vi "AutonVisionTrack.vi"(3 "Refnum in":refnum<k33>) -> (10 "rt fifo out":refnum<k33>)   [LabVIEW 2014]
uses:
  TeleopCmd.ctl
  CmdFlag.ctl
  VisionInfoCluster.ctl
  AutonCals.vi
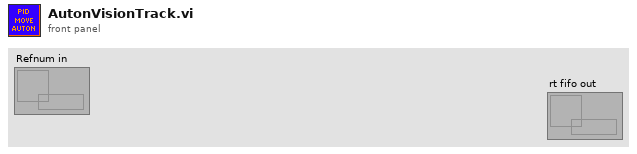
[diagram p1: front panel]
types:
  T1 = typedef "VisionInfoCluster.ctl" = cluster{"X":dbl, "Y":dbl}
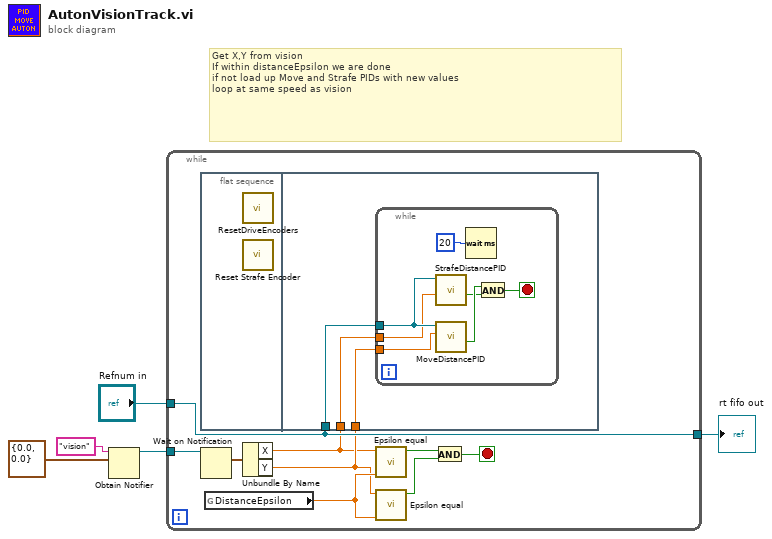
[diagram p0: block diagram]
diagram:
  # "Get X,Y from vision\nIf within distanceEpsilon we are done\nif not load up Move and Strafe PIDs with new values\nloop at same speed as vision"
  n1 = Obtain Notifier(name (unnamed)="vision", notification data type=T1 {"X"=0.0, "Y"=0.0}) -> (notifier out=w3:refnum<notifier>)  [unwired: 2 in, 2 out]
  n2 = while {
    tunnel: w3 -> [w11]
    tunnel: "Refnum in" -> [w8]
    tunnel: [w8] -> w1
    stop <- w12 stop-if-true
    n3 = flat-sequence {
      tunnel: w8 -> [w17]
      tunnel: w7 -> [w16]
      tunnel: w6 -> [w15]
      frame #0 {
        n4 = call "ResetDriveEncoders.vi"() -> ()  [unwired: 12 in]
        n5 = call "Reset Strafe Encoder.vi"() -> ()  [unwired: 12 in]
      }
      frame #1 {
        n6 = while {
          tunnel: w17 -> [w20]
          tunnel: w16 -> [w19]
          tunnel: w15 -> [w18]
          stop <- w24 stop-if-true
          n7 = call "StrafeDistancePID.vi"("Distance"=w18, "Refnum in"=w20) -> ("Boolean"=w22:bool)  [unwired: 7 in, 2 out]
          n8 = call "MoveDistancePID.vi"("Distance"=w19, "Refnum in"=w20) -> ("Boolean"=w23:bool)  [unwired: 7 in, 2 out]
          n9 = Wait (ms)(milliseconds to wait=u32 20) -> ()  [unwired: 1 out]
          n10 = And(x=w23, y=w22) -> (x .and. y?=w24:bool)
        }
      }
    }
    n11 = Wait on Notification(notifier=w11) -> (notification=w10:T1)  [unwired: 3 in, 3 out]
    n12 = global read "AutonCals.vi" "DistanceEpsilon"() -> (w9:dbl)
    n13 = Unbundle By Name(w10) -> ("X"=w6:dbl, "Y"=w7:dbl)
    n14 = call "Epsilon equal.vi"("Epsilon"=w9, "Value1"=w6) -> ("Boolean"=w13:bool)  [unwired: 9 in]
    n15 = call "Epsilon equal.vi"("Epsilon"=w9, "Value1"=w7) -> ("Boolean"=w14:bool)  [unwired: 9 in]
    n16 = And(x=w13, y=w14) -> (x .and. y?=w12:bool)
  }
  "rt fifo out" <- w1
